vi "GetCurrentCharacter.vi"(8 "error in (no error)":errorcluster, 11 "PathTokenizer in":refnum<class "PathTokenizer.lvclass">) -> (0 "error out":errorcluster, 2 "Current Character":string, 3 "PathTokenizer out":refnum<class "PathTokenizer.lvclass">)   [LabVIEW 2019, in "PathTokenizer.lvclass"]
uses:
  PathTokenizer.lvclass
  PathTokenizer.lvclass/PathTokenizer.ctl
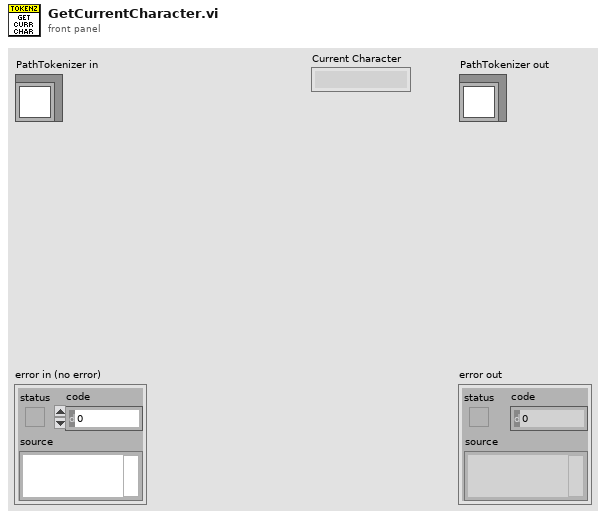
[diagram p1: front panel]
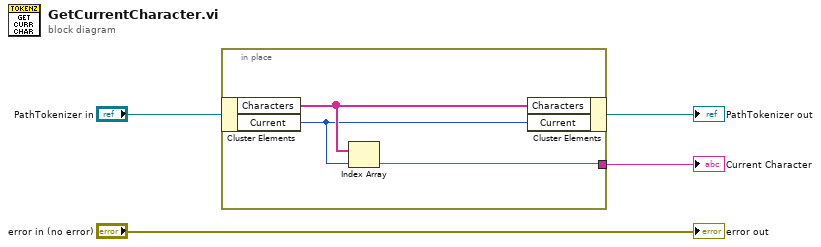
[diagram p0: block diagram]
diagram:
  n1 = in-place "In Place Element Structure" {
    in-place-border: [w5] -> w2
    n2 = in-place-cluster #1("PathTokenizer in") -> ("Characters"=w7:string[], "Current"=w6:i32)
    n3 = Index Array(array=w7, index=w6) -> (element=w5:string)
    n4 = in-place-cluster #1("Characters"=w7, "Current"=w6) -> (→"PathTokenizer out":refnum<class "PathTokenizer.lvclass">)
  }
  "Current Character" <- w2
  "error out" <- "error in (no error)"
